vi "ODE Linear nth Order Symbolic.vi"(2 "X0":dbl[](array[numeric]) format="%.1f", 3 "A (a0,a1,...an-1)":dbl[](array[numeric]) format="%.1f") -> (0 "error":i32, 1 "formula":string=" ")   [LabVIEW 2020, in "NI_Gmath.lvlib"]
doc: "Solves an nth-order, homogeneous linear differential equation with constant coefficients in symbolic form."
uses:
  NI_Gmath.lvlib
  Complex A x Vector.vi
  Polynomial Roots (DBL).vi
  Complex Inverse Matrix.vi
  NI_AALBase.lvlib
  NI_AALPro.lvlib
panel:
  # "Example:\n\n A: 1.1 and 2.0 and -7.3 \n X0: 1.0 and 2.4 and -1.4"
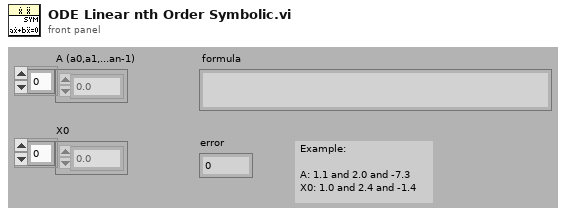
[diagram p1: front panel]
types:
  T1 = typedef "NI_Matrix.lvlib/ComplexMatrix.ctl" = cdb[][]
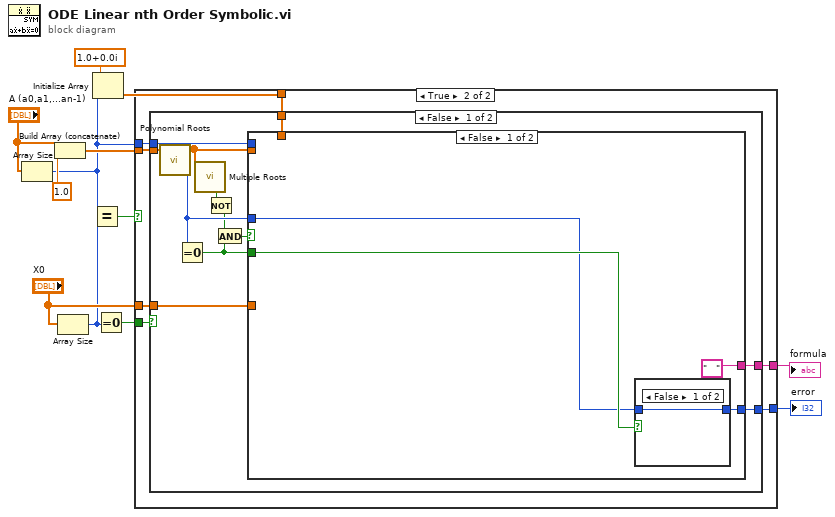
[diagram p0: block diagram]
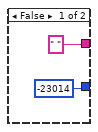
[diagram p2: hidden frame]
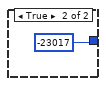
[diagram p3: hidden frame]
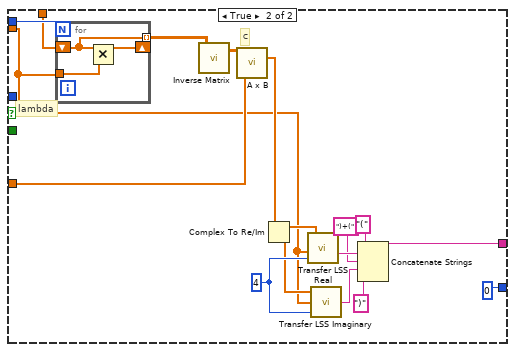
[diagram p4: hidden frame]
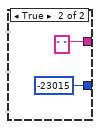
[diagram p5: hidden frame]
diagram:
  n1 = Array Size(array="A (a0,a1,...an-1)") -> (size(s)=w3:i32)
  n2 = Build Array (concatenate)("A (a0,a1,...an-1)", 1.0) -> (w6:dbl[])
  n3 = Array Size(array="X0") -> (size(s)=w8:i32)
  n4 = Equal?(x=w3, y=w8) -> (x = y?=w12:bool)
  n5 = Initialize Array(cdb 1.0+0.0i, w3) -> (w1:cdb[])
  n6 = Equal To 0?(x=w8) -> (x = 0?=w10:bool)
  n7 = case shown="True" w12 {
    tunnel: [-23014 w20] -> w11
    tunnel: w10 -> [_ w21]
    tunnel: w6 -> [_ w19]
    tunnel: "X0" -> [_ w18]
    tunnel: w3 -> [_ w17]
    tunnel: [" " w16] -> w7
    tunnel: w1 -> [_ w15]
    frame False {
    }
    frame True {
      n8 = case shown="False" w21 {
        tunnel: [w33 -23015] -> w20
        tunnel: w19 -> [w32 _]
        tunnel: w18 -> [w31 _]
        tunnel: w17 -> [w29 _]
        tunnel: [w28 " "] -> w16
        tunnel: w15 -> [w22 _]
        frame False {
          n9 = call-poly "Polynomial Roots.vi"("P(x)"=w32) -> ("error"=w30:i32, "Roots"=w27:cdb[])  [unwired: 9 in]
          n10 = Equal To 0?(x=w30) -> (x = 0?=w23:bool)
          n11 = call "Multiple Roots.vi"("Polynomial Roots"=w27) -> ("multiple roots"=w26:bool)
          n12 = Not(x=w26) -> (.not. x?=w25:bool)
          n13 = And(x=w25, y=w23) -> (x .and. y?=w24:bool)
          n14 = case shown="False" w24 {
            tunnel: w27 -> [_ w41]
            tunnel: w31 -> [_ w54]
            tunnel: [w34 0] -> w33
            tunnel: w30 -> [w35 _]
            tunnel: w29 -> [_ w43]
            tunnel: ["   " w49] -> w28
            tunnel: w23 -> [w36 _]
            tunnel: w22 -> [_ w42]
            frame False {
              n15 = case shown="False" w36 {
                tunnel: w35 -> [w38 _]
                tunnel: [w38 -23017] -> w34
                frame False {
                }
                frame True {
                }
              }
            }
            frame True {
              w53 = u32 4
              # "lambda"
              # "C"
              n16 = for {
                N: w43 -> [_]
                tunnel: w41 -> [w59]
                shift-right: [w58] -> _
                shift-left: w42 -> [w57]
                tunnel: [w57] -> w40 mode=indexing
                n17 = Multiply(x=w57, y=w59) -> (x*y=w58:cdb[])
              }
              n18 = call-poly "Inverse Matrix.vi"("Input Matrix"=w40) -> ("Inverse Matrix"=w55:T1)  [unwired: 1 in, 1 out]
              n19 = call-poly "A x B.vi"("Vector"=w54, "A"=w55) -> ("A x Vector"=w52:cdb[])  [unwired: 1 out]
              n20 = Complex To Re/Im(x + iy=w52) -> (x=w51:dbl[], y=w50:dbl[])
              n21 = call "Transfer LSS Real.vi"("precision"=w53, "lambda"=w41, "beta"=w51) -> ("formula linear combination"=w47:string)
              n22 = call "Transfer LSS Imaginary.vi"("precision"=w53, "lambda"=w41, "beta"=w50) -> ("formula linear combination"=w45:string)
              n23 = Concatenate Strings("(", w47, ")+(", w45, ")") -> (w49:string)
            }
          }
        }
        frame True {
        }
      }
    }
  }
  "error" <- w11
  "formula" <- w7
